vi "Launch Async Loop.vi"(8 "error in (no error)":errorcluster, 11 "Input Data":T1) -> (0 "error out":errorcluster)   [LabVIEW 2015, in "Shared Variable Custom Device.lvlib"]
doc: "Launches the Async Loop with call and forget."
uses:
  Shared Variable Custom Device.lvlib
  Input Data Control.ctl
  <vilib>/Utility/VariantDataType/Type.ctl
  Aync Communication.vi
  <vilib>/Utility/VariantDataType/VariantType.lvlib
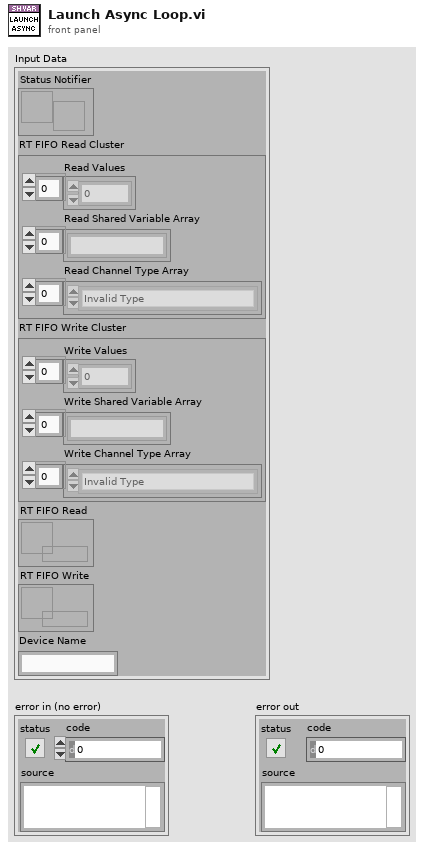
[diagram p1: front panel]
types:
  T1 = typedef "Shared Variable Custom Device.lvlib/Input Data Control.ctl" = cluster{"Status Notifier":refnum<notifier>, "RT FIFO Read Cluster":cluster{"Read Values":dbl[], "Read Shared Variable Array":string[], "Read Channel Type Array":T2[]}, "RT FIFO Write Cluster":cluster{"Write Values":dbl[], "Write Shared Variable Array":string[], "Write Channel Type Array":T2[]}, "RT FIFO Read":refnum<k33>, "RT FIFO Write":refnum<k33>, "Device Name":string}
  T2 = typedef "VariantType.lvlib/Type.ctl" = enum8{"Invalid Type", "Void", "I8", "I16", "I32", "I64", "U8", "U16", "U32", "U64", "Single Float", "Double Float", "Extended Float", "Single Complex", "Double Complex", "Extended Complex", "Enum U8", "Enum U16", "Enum U32", "Enum U64", "Single Float With Unit", "Double Float With Unit", "Extended Float With Unit", "Single Complex with Unit", "Double Complex with Unit", "Extended Complex with Unit", "Boolean", "String", "Path", "Picture", "Tag", "Array", "Cluster", "Variant", "LV Variant", "Waveform", "Timestamp", "Digital Waveform", "Digital Data", "ExpressData", "Refnum", "External Data", "VI", "Poly VI", "LabVIEW Class Instance", "Fixed Point"}
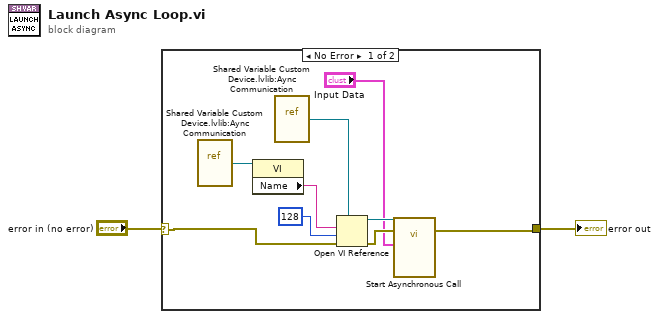
[diagram p0: block diagram]
diagram:
  n1 = case shown="No Error" "error in (no error)" {
    selector: "error in (no error)" -> [w9 w12]
    tunnel: [w3 w12] -> w2
    frame No Error {
      n2 = vi-ref "Shared Variable Custom Device.lvlib:Aync Communication.vi"() -> (w8:refnum<vi>)
      n3 = property class="VI"(reference=w8) -> ("Name"=w11:string)  [unwired: 1 in, 2 out]
      n4 = vi-ref "Shared Variable Custom Device.lvlib:Aync Communication.vi"() -> (w7:refnum<vi>)
      n5 = Open VI Reference(type specifier VI Refnum (for type only)=w7, vi path=w11, options=128, error in (no error)=w9) -> (vi reference=w6:refnum<vi>, error out=w5:errorcluster)  [unwired: 2 in]
      n6 = call-by-ref "Start Asynchronous Call"(reference=w6, error in=w5, "Input Data"="Input Data") -> (error out=w3:errorcluster)  [unwired: 11 in, 1 out]
    }
    frame Error {
    }
  }
  "error out" <- w2
